vi "10.2 Low level writing and reading data to a file.vi"() -> ()   [LabVIEW 2019]
panel:
  in  "Number of samples":i32
  out "Message":string
  in  "Sample Rate":dbl
  in  "User name":string
  out "Format into string":string
  in  "Precision":i16
  out "F-format string":string
  in  "Stop":bool
  in  "File Path Control":path
  # "NUMBER INTO STRING"
  # "MULTIPLE ITEMS AND DATA TYPES INTO STRING"
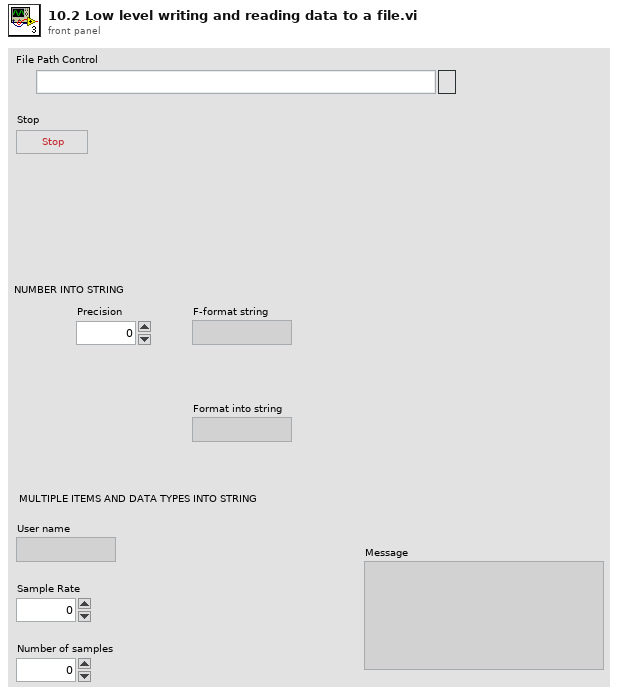
[diagram p1: front panel]
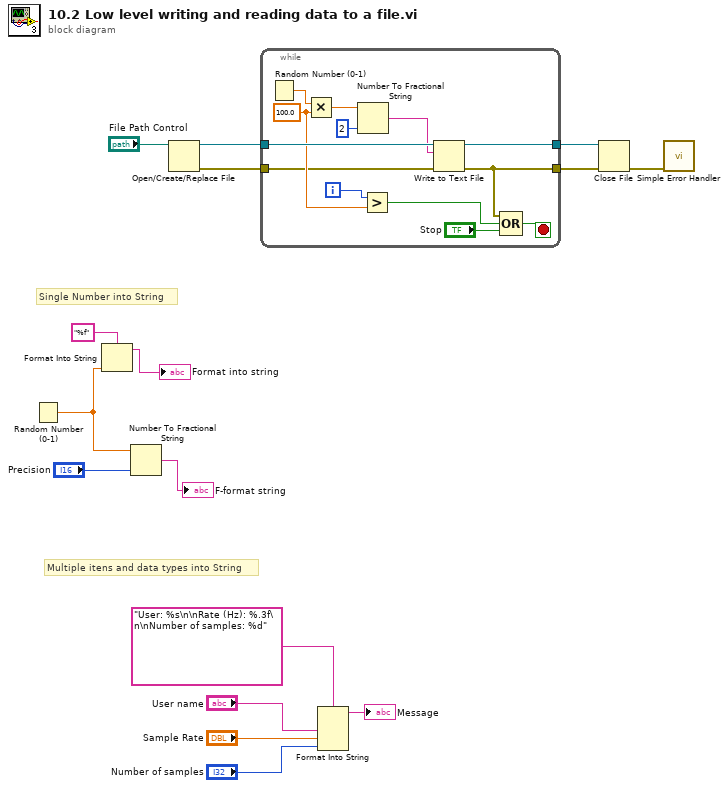
[diagram p0: block diagram]
diagram:
  # "Multiple itens and data types into String"
  # "Single Number into String"
  n1 = Random Number (0-1)() -> (number: 0 to 1=w9:dbl)
  n2 = Format Into String "Format Into String"(format string="%f", w9) -> (resulting string=→"Format into string":string)  [unwired: 2 in, 1 out]
  n3 = Number To Fractional String(number=w9, precision (6)="Precision") -> (F-format string=→"F-format string":string)  [unwired: 2 in]
  n4 = Open/Create/Replace File(file path (use dialog)="File Path Control") -> (refnum out=w13:refnum<file>, error out=w6:errorcluster)  [unwired: 5 in, 1 out]
  n5 = while {
    tunnel: w6 -> [w20]
    tunnel: [w22] -> w16
    tunnel: w13 -> [w29]
    tunnel: [w28] -> w12
    i -> [w23]
    stop <- w27 stop-if-true
    w24 = 100.0 ("y")
    n6 = Random Number (0-1)() -> (number: 0 to 1=w25:dbl)
    n7 = Multiply(x=w25, y=w24) -> (x*y=w19:dbl)
    n8 = Number To Fractional String(number=w19, precision (6)=i16 2) -> (F-format string=w17:string)  [unwired: 2 in]
    n9 = Greater?(x=w23, y=w24) -> (0:w21:bool)
    n10 = Write to Text File(file (use dialog)=w29, text=w17, error in=w20) -> (refnum out=w28:refnum<file>, error out=w22:errorcluster)  [unwired: 1 in, 1 out]
    n11 = Compound Arithmetic op=OR(w22, w21, "Stop") -> (w27:bool)
  }
  n12 = Format Into String "Format Into String"(format string="User: %s\n\nRate (Hz): %.3f\n\nNumber of samples: %d", "User name", "Sample Rate", "Number of samples") -> (resulting string=→"Message":string)  [unwired: 2 in, 1 out]
  n13 = Close File(refnum=w12, error in=w16) -> (error out=w15:errorcluster)  [unwired: 1 out]
  n14 = call <vilib>:"Simple Error Handler.vi"("error in (no error)"=w15) -> ()  [unwired: 4 in, 5 out]
